vi "Create Windows Shortcut.vi"(6 "Icon Location (0)":i32, 7 "Arguments (none)":string, 8 "error in (no error)":errorcluster, 9 "Shortcut Name (empty)":string, 10 "Shortcut Folder (empty)":path, 11 "Target Path (empty)":path) -> (0 "error out":errorcluster)   [LabVIEW 2011]
panel:
  in  "IWshRuntimeLibrary.IWshShortcut":refnum<k7>
  in  "IWshRuntimeLibrary.IWshShell3":refnum<k7>
  # "Shortcut Properties:\n\n*  Start In = Target Folder\n*  No shortcut key\n*  Normal window\n*  Icon of Target,0\n*  No comment"
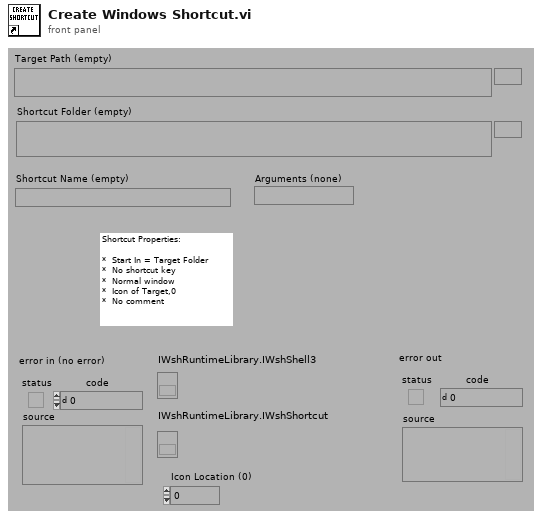
[diagram p1: front panel]
types:
  T1 = cluster{"Arguments":string, "Description":string, "Hotkey":string, "IconLocation":string, "TargetPath":string, "WindowStyle":i32, "WorkingDirectory":string}
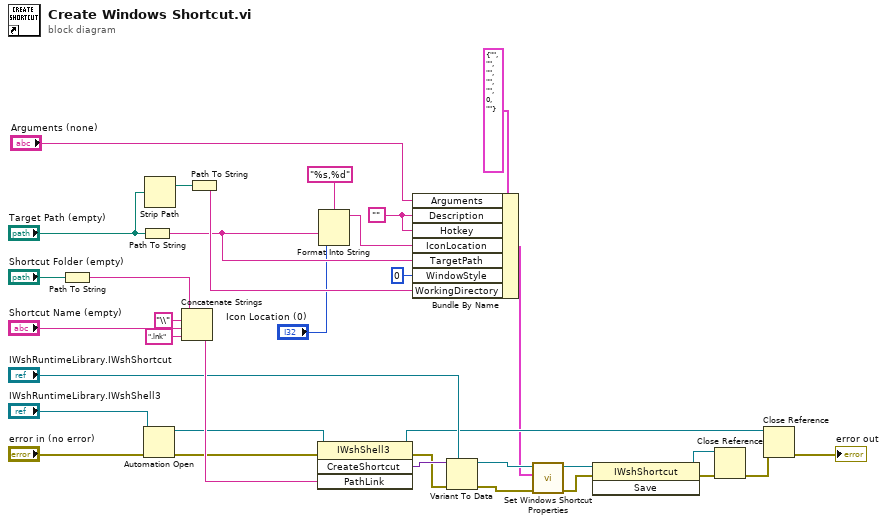
[diagram p0: block diagram]
diagram:
  w10 = ""
  n1 = Path To String(path="Shortcut Folder (empty)") -> (string=w24:string)
  n2 = Path To String(path="Target Path (empty)") -> (string=w3:string)
  n3 = Automation Open(error in (no error)="error in (no error)", Automation Refnum="IWshRuntimeLibrary.IWshShell3") -> (Automation Refnum=w26:refnum<k7>, error out=w27:errorcluster)  [unwired: 2 out]
  n4 = Strip Path(path="Target Path (empty)") -> (stripped path=w8:path)  [unwired: 1 out]
  n5 = Concatenate Strings(w24, "\\" ("Substring"), "Shortcut Name (empty)", ".lnk" ("Substring")) -> (w28:string)
  n6 = Path To String(path=w8) -> (string=w7:string)
  n7 = invoke class="IWshShell3" method="CreateShortcut"(reference=w26, error in=w27, "PathLink"=w28) -> (reference out=w18:refnum<k7>, error out=w31:errorcluster, "CreateShortcut"=w32:variant)  [unwired: 1 in, 1 out]
  n8 = Format Into String(format string="%s,%d", w3, "Icon Location (0)") -> (resulting string=w1:string)  [unwired: 2 in, 1 out]
  n9 = Bundle By Name(cluster=T1 {"Arguments"="", "Description"="", "Hotkey"="", "IconLocation"="", "TargetPath"="", "WindowStyle"=0, "WorkingDirectory"=""} ("Shortcut Options"), "Arguments"="Arguments (none)", "Description"=w10, "Hotkey"=w10, "IconLocation"=w1, "TargetPath"=w3, "WindowStyle"=0, "WorkingDirectory"=w7) -> (w11:T1)
  n10 = Variant To Data(error in=w31, type="IWshRuntimeLibrary.IWshShortcut", Variant=w32) -> (data=w16:refnum<k7>, error out=w14:errorcluster)
  n11 = call "Set Windows Shortcut Properties.vi"("error in"=w14, "Shortcut Options"=w11, "IWshRuntimeLibrary.IWshShortcut"=w16) -> ("error out"=w13:errorcluster, "dup IWshRuntimeLibrary.IWshShortcut"=w15:refnum<k7>)  [unwired: 3 out]
  n12 = invoke class="IWshShortcut" method="Save"(reference=w15, error in=w13) -> (reference out=w21:refnum<k7>, error out=w20:errorcluster)  [unwired: 1 in, 1 out]
  n13 = Close Reference(reference=w21, error in (no error)=w20) -> (error out=w19:errorcluster)
  n14 = Close Reference(reference=w18, error in (no error)=w19) -> (error out=→"error out":errorcluster)
